vi "Connect_to_BSA_IP.vi"() -> (0 "error out":errorcluster, 1 "BSA":refnum<k7>)   [LabVIEW 2014]
uses:
  Globals/LDA_meas_global_1.vi
panel:
  out "First error":errorcluster
  in  "BSACtrl.IBSA":refnum<k7>
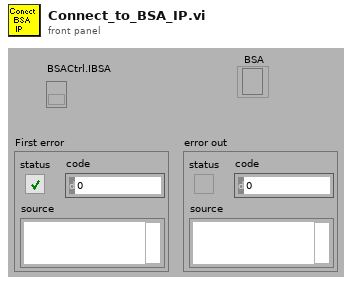
[diagram p1: front panel]
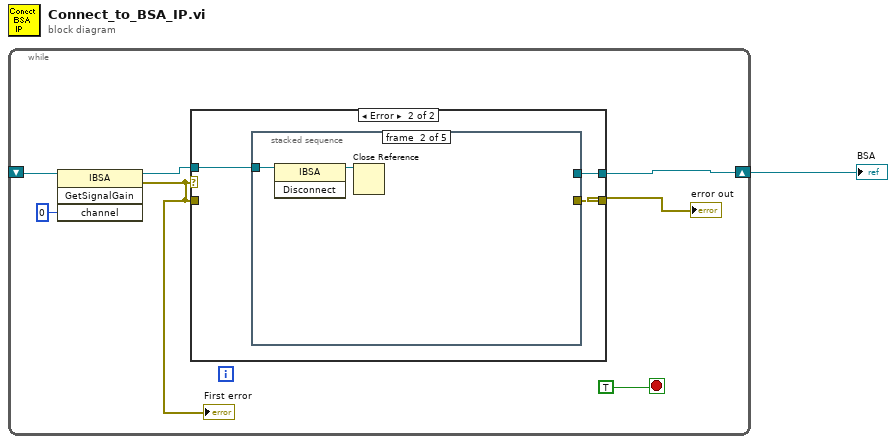
[diagram p0: block diagram]
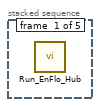
[diagram p3: hidden frame]
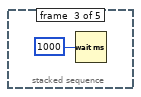
[diagram p4: hidden frame]
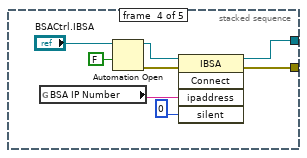
[diagram p5: hidden frame]
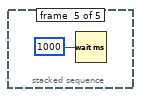
[diagram p6: hidden frame]
diagram:
  n1 = while {
    shift-right: [w4] -> w1
    shift-left: _ -> [w5]
    stop <- TRUE stop-if-true
    n2 = invoke class="IBSA" method="GetSignalGain"(reference=w5, "channel"=0) -> (reference out=w6:refnum<k7>, error out=w7:errorcluster)  [unwired: 2 in, 2 out]
    "First error" <- w7
    n3 = case shown="Error" w7 {
      tunnel: [w10 w13] -> w4
      tunnel: w6 -> [w10 w11]
      tunnel: [w9 w12] -> w3
      tunnel: w7 -> [w9 _]
      frame No Error {
      }
      frame Error {
        n4 = stacked-sequence {
          tunnel: w11 -> [_ w15 _ _ _]
          tunnel: [_ _ _ w18 _] -> w13
          tunnel: [_ _ _ w17 _] -> w12
          frame #0 {
            n5 = call "Run_EnFlo_Hub.vi"() -> ()  [unwired: 8 out]
          }
          frame #1 {
            n6 = invoke class="IBSA" method="Disconnect"(reference=w15) -> (reference out=w14:refnum<k7>)  [unwired: 2 in, 2 out]
            n7 = Close Reference(reference=w14) -> ()  [unwired: 1 in, 1 out]
          }
          frame #2 {
            n8 = Wait (ms)(milliseconds to wait=u32 1000) -> ()  [unwired: 1 out]
          }
          frame #3 {
            n9 = global read "LDA_meas_global_1.vi" "BSA IP Number"() -> (w20:string)
            n10 = Automation Open(Automation Refnum="BSACtrl.IBSA", 9:FALSE ("open new instance (false)")) -> (Automation Refnum=w23:refnum<k7>, error out=w22:errorcluster)  [unwired: 2 in]
            n11 = invoke class="IBSA" method="Connect"(reference=w23, error in=w22, "ipaddress"=w20, "silent"=0) -> (reference out=w18:refnum<k7>, error out=w17:errorcluster)  [unwired: 1 in, 3 out]
          }
          frame #4 {
            n12 = Wait (ms)(milliseconds to wait=u32 1000) -> ()  [unwired: 1 out]
          }
        }
      }
    }
    "error out" <- w3
  }
  "BSA" <- w1
